vi "Slider value change event reducer.vi"(9 "Ignore delta sec":dbl=0.5 caption="Time Target (s)", 11 "Event Type":T1) -> (2 "Process event?":bool)   [LabVIEW 2013]
doc: "This vi is be placed inside Event Structure cases for a slider with 2 events: value change and mouse up events. It is used to reduce the number of events normally generated when user holds down the slider and moves it, which can easily be 10 or 20 events per second. This vi, which is reentrant so it can be used in multiple instances, has an internal timer and the output \"process event?\" is true if (first call OR time elapsed OR event type = mouse up."
uses:
  <vilib>/event_ctls.llb/lveventtype.ctl
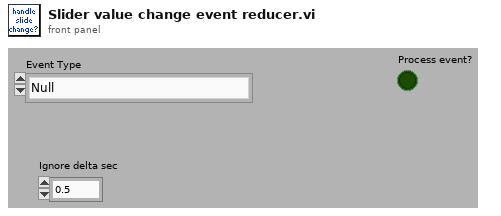
[diagram p1: front panel]
types:
  T1 = typedef "lveventtype.ctl" = enum32{"Null", "Timeout", "Annotation Menu Selection", "Annotation Menu Selection?", "App Instance Close", "App Instance Close?", "Autoscale Range Change", "Bookmark Info Change", "Cell Edit", "Cell Edit?", "Cursor Grab", "Cursor Grab?", "Cursor Menu Selection", "Cursor Menu Selection?", "Cursor Move", "Cursor Release", "Data Change", "Direction Change", "Display State Change", "Drag Ended", "Drag Enter", "Drag Leave", "Drag Over", "Drag Source Update", "Drag Starting", "Drag Starting?", "Drop", "Exec State Change", "Key Down", "Key Down?", "Key Repeat", "Key Repeat?", "Key Up", "Listbox Double Click", "Menu Activation?", "Menu Selection (App)", "Menu Selection? (App)", "Menu Selection (User)", "Mouse Down", "Mouse Down?", "Mouse Enter", "Mouse Leave", "Mouse Move", "Mouse Up", "Mouse Wheel", "NI Security User Change (App)", "Pane Size", "Panel Close", "Panel Close?", "Panel Resize", "Plot Attribute Change", "Scale Range Change", "Shortcut Menu Activation?", "Shortcut Menu Selection (App)", "Shortcut Menu Selection? (App)", "Shortcut Menu Selection (User)", "Tree Double Click", "Tree Drag", "Tree Drag?", "Tree Drop", "Tree Drop?", "Tree Item Close", "Tree Item Close?", "Tree Item Open", "Tree Item Open?", "User Event", "Value Change"}
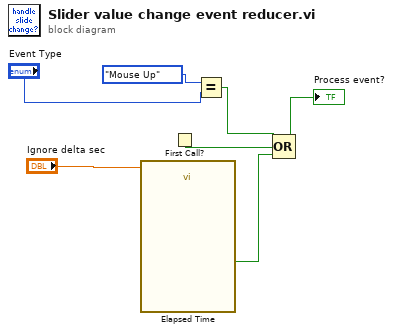
[diagram p0: block diagram]
diagram:
  n1 = call "Elapsed Time"("Time Target (s)"="Ignore delta sec") -> ("Time has Elapsed"=w6:bool)  [unwired: 11 in, 7 out]
  n2 = First Call?() -> (First Call?: T/F=w5:bool)
  n3 = Equal?(x=lveventtype."Mouse Up", y="Event Type") -> (x = y?=w4:bool)
  n4 = Compound Arithmetic op=OR(w4, w5, w6) -> (→"Process event?":bool)
